vi "Read Client Configuration.vi"(8 "error in (no error)":errorcluster, 11 "Configuration File Path":path) -> (0 "error out":errorcluster, 3 "Client Configuration":T1)   [LabVIEW 2024]
doc: "Reads the client configuration from the configuration file."
uses:
  Controls/Client/Client Configuration.ctl
  <vilib>/Utility/config.llb/Read Key (String).vi
  <vilib>/Utility/config.llb/NI_LVConfig.lvlib
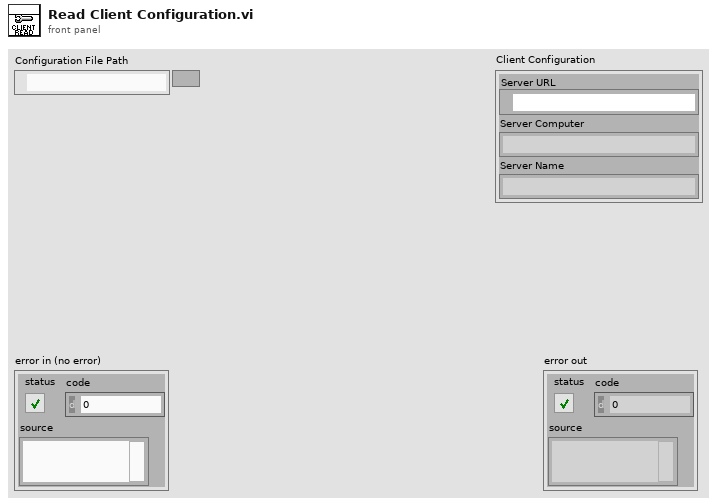
[diagram p1: front panel]
types:
  T1 = typedef "Client Configuration.ctl" = cluster{"Server URL":refnum<k21>, "Server Computer":string, "Server Name":string}
  T2 = typedef "NI_LVConfig.lvlib/Config Data RefNum.ctl" = refnum<k1>
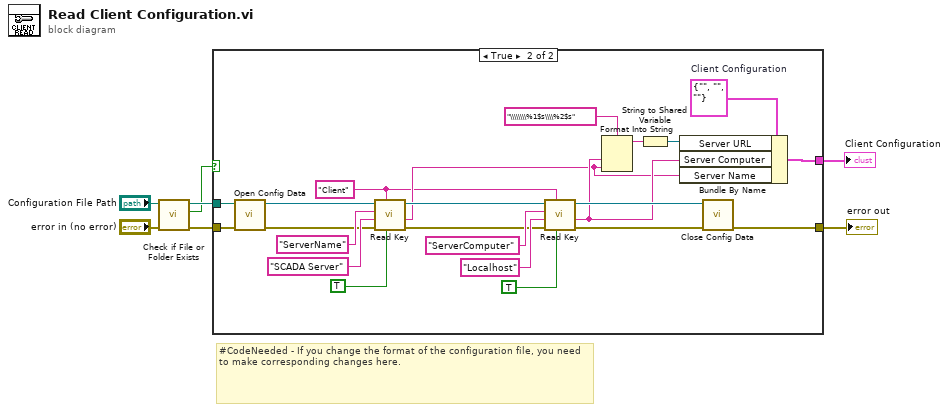
[diagram p0: block diagram]
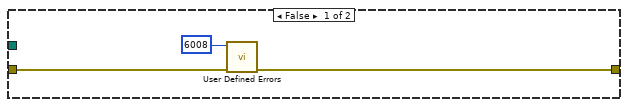
[diagram p2: hidden frame]
diagram:
  # "#CodeNeeded - If you change the format of the configuration file, you need to make corresponding changes here."
  n1 = call <vilib>:"Check if File or Folder Exists.vi"("error in (no error)"="error in (no error)", "path"="Configuration File Path") -> ("error out"=w2:errorcluster, "file or folder exists?"=w1:bool, "dup path"=w4:path)  [unwired: 7 in]
  n2 = case shown="True" w1 {
    tunnel: [w9 w33] -> w7
    tunnel: [_ w32] -> w6
    tunnel: w4 -> [_ w20]
    tunnel: w2 -> [w8 w19]
    frame False {
      n3 = call "User Defined Errors.vi"("error in (no error)"=w8, "Error Code (0)"=6008 ("error code (0)")) -> ("error out"=w9:errorcluster)  [unwired: 9 in]
    }
    frame True {
      w13 = T1 {"Server URL"="", "Server Computer"="", "Server Name"=""}  # Client Configuration
      w11 = "Client" ("section")
      n4 = call <vilib>:"Open Config Data.vi"("error in (no error)"=w19, "configuration file path"=w20) -> ("error out"=w21:errorcluster, "refnum"=w22:T2)  [unwired: 7 in, 1 out]
      n5 = call-poly <vilib>:"Read Key.vi"("read raw string? (F)"=TRUE, "section"=w11, "error in (no error)"=w21, "default value"="SCADA Server", "key"="ServerName", "refnum"=w22) -> ("error out"=w25:errorcluster, "value"=w12:string, "refnum out"=w26:T2)  [unwired: 2 in, 1 out]
      n6 = call-poly <vilib>:"Read Key.vi"("read raw string? (F)"=TRUE, "section"=w11, "error in (no error)"=w25, "default value"="Localhost", "key"="ServerComputer", "refnum"=w26) -> ("error out"=w23:errorcluster, "value"=w15:string, "refnum out"=w24:T2)  [unwired: 2 in, 1 out]
      n7 = Format Into String(format string="\\\\\\\\%1$s\\\\%2$s", w15, w12) -> (resulting string=w16:string)  [unwired: 2 in, 1 out]
      n8 = String to Shared Variable(0:w16) -> (2:w29:refnum<k21>)  [unwired: 1 out]
      n9 = Bundle By Name(cluster=w13, "Server URL"=w29, "Server Computer"=w15, "Server Name"=w12) -> (w32:T1)
      n10 = call <vilib>:"Close Config Data.vi"("error in (no error)"=w23, "refnum"=w24) -> ("error out"=w33:errorcluster)  [unwired: 8 in, 1 out]
    }
  }
  "error out" <- w7
  "Client Configuration" <- w6
